vi "Eval y=f(a,x).vi"(4 "number of points":u32=10, 5 "formula":string, 6 "Parameters":cluster{"name":string, "value":dbl}[](array[cluster]) {"value" format="%.2f"}, 7 "end":dbl=1.0 format="%.2f", 8 "start":dbl format="%.2f") -> (0 "error":i32, 1 "ticks":u32, 2 "Y":dbl[](array[numeric]) format="%.2f", 3 "X":dbl[](array[numeric]) format="%.2f")   [LabVIEW 2020, in "NI_Gmath.lvlib"]
doc: "A generalized version of the Eval y=f(x) VI with the possibility of adding some parameters into the formula."
uses:
  <vilib>/gmath/NI_Gmath.lvlib
panel:
  # "Example:\n\n number of points: 100 \n start: 0.0\n end: 1.0\n Parameters: (a,1) and (b,2) \n formula: sin(t*a)+b"
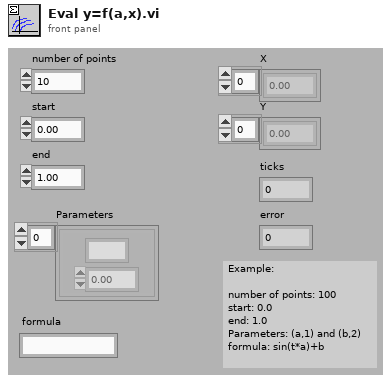
[diagram p1: front panel]
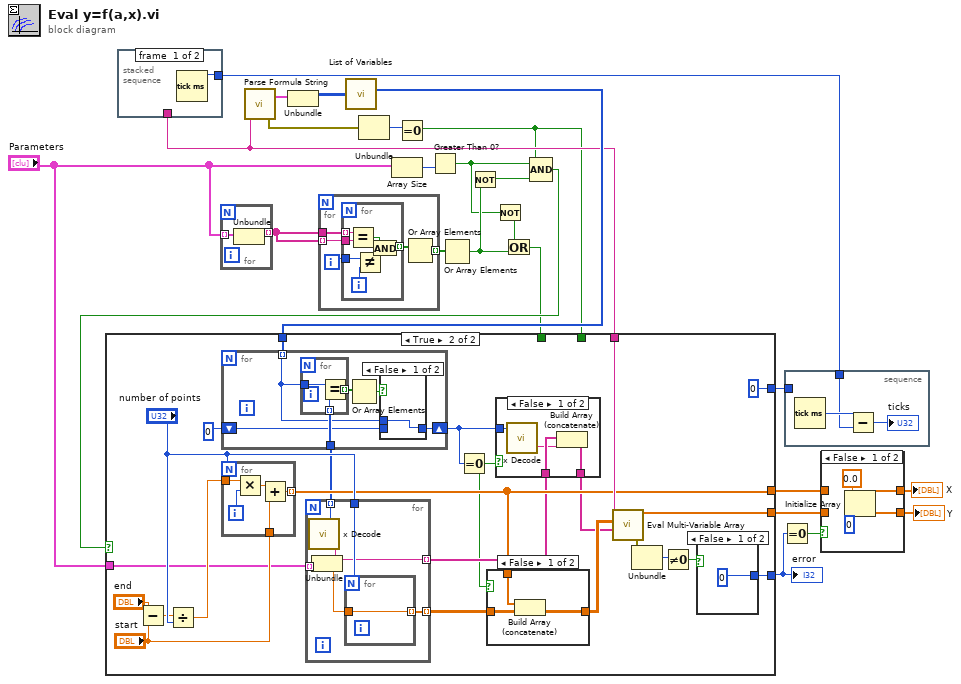
[diagram p0: block diagram]
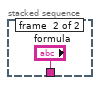
[diagram p3: hidden frame]
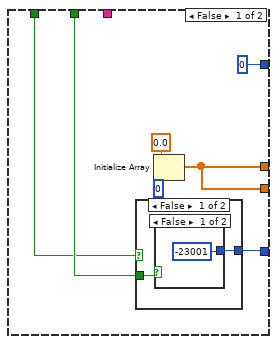
[diagram p4: hidden frame]
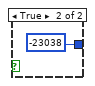
[diagram p5: hidden frame]
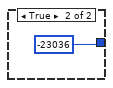
[diagram p6: hidden frame]
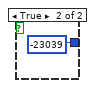
[diagram p10: hidden frame]
diagram:
  n1 = stacked-sequence {
    tunnel: [w26 _] -> w24
    tunnel: [_ "formula"] -> w4
    frame #0 {
      n2 = Tick Count (ms)() -> (millisecond timer value=w26:u32)
    }
    frame #1 {
    }
  }
  n3 = for {
    tunnel: "Parameters" -> [w29] mode=indexing
    tunnel: [w28] -> w12 mode=indexing
    n4 = Unbundle(w29) -> ("name"=w28:string)  [unwired: 1 out]
  }
  n5 = call <vilib>:"Parse Formula String.vi"("formula"=w4) -> ("error out"=w23:errorcluster, "Parsed Formula"=w15:cluster{"Table":i32[][], "Y Values":dbl[]})  [unwired: 1 in]
  n6 = Unbundle(w15) -> ("Table"=w14:i32[][])  [unwired: 1 out]
  n7 = for {
    tunnel: w12 -> [w34]
    tunnel: w12 -> [w33] mode=indexing
    tunnel: [w30] -> w11 mode=indexing
    i -> [w32]
    n8 = for {
      tunnel: w34 -> [w41] mode=indexing
      tunnel: w33 -> [w40]
      tunnel: w32 -> [w39]
      tunnel: [w35] -> w31 mode=indexing
      i -> [w38]
      n9 = Equal?(x=w41, y=w40) -> (x = y?=w37:bool)
      n10 = Not Equal?(x=w39, y=w38) -> (x != y?=w36:bool)
      n11 = And(x=w37, y=w36) -> (x .and. y?=w35:bool)
    }
    n12 = Or Array Elements(Boolean array=w31) -> (logical OR=w30:bool)
  }
  n13 = call <vilib>:"List of Variables.vi"("Table"=w14) -> ("List of variables"=w13:i32[])
  n14 = Unbundle(w23) -> ("code"=w22:i32)  [unwired: 2 out]
  n15 = Array Size(array="Parameters") -> (size(s)=w9:i32)
  n16 = Equal To 0?(x=w22) -> (x = 0?=w3:bool)
  n17 = Greater Than 0?(x=w9) -> (x > 0?=w7:bool)
  n18 = Or Array Elements(Boolean array=w11) -> (logical OR=w8:bool)
  n19 = Not(x=w8) -> (.not. x?=w10:bool)
  n20 = Not(x=w7) -> (.not. x?=w5:bool)
  n21 = Or(x=w5, y=w8) -> (x .or. y?=w2:bool)
  n22 = Compound Arithmetic op=AND(w3, w7, w10) -> (w6:bool)
  n23 = case shown="True" w6 {
    tunnel: w4 -> [_ w76]
    tunnel: [w45 w69] -> w19
    tunnel: [w45 w68] -> w17
    tunnel: [0 0] -> w25
    tunnel: [w44 w62] -> w21
    tunnel: w13 -> [_ w61]
    tunnel: "Parameters" -> [_ w58]
    tunnel: w3 -> [w43 _]
    tunnel: w2 -> [w42 _]
    frame False {
      n24 = case shown="False" w42 {
        tunnel: [w50 -23036] -> w44
        tunnel: w43 -> [w49 _]
        frame False {
          n25 = case shown="False" w49 {
            tunnel: [-23001 -23038] -> w50
            frame False {
            }
            frame True {
            }
          }
        }
        frame True {
        }
      }
      n26 = Initialize Array(0.0, 0) -> (w45:dbl[])
    }
    frame True {
      n27 = Subtract(x="end", y="start") -> (x-y=w70:dbl)
      n28 = Divide(x=w70, y="number of points") -> (x/y=w71:dbl)
      n29 = for {
        N: "number of points" -> [_]
        tunnel: w71 -> [w103]
        tunnel: "start" -> [w99]
        tunnel: [w100] -> w69 mode=indexing
        i -> [w102]
        n30 = Multiply(x=w103, y=w102) -> (x*y=w101:dbl)
        n31 = Add(x=w101, y=w99) -> (x+y=w100:dbl)
      }
      n32 = for {
        tunnel: w58 -> [w109] mode=indexing
        tunnel: [w105] -> w57 mode=indexing
        tunnel: "number of points" -> [w108]
        tunnel: [w106] -> w75 mode=indexing
        tunnel: [w104] -> w60 mode=indexing
        n33 = Unbundle(w109) -> ("name"=w105:string, "value"=w107:dbl)
        n34 = call <vilib>:"x Decode.vi"("x string"=w105) -> ("number"=w104:i32)  [unwired: 1 in, 1 out]
        n35 = for {
          N: w108 -> [_]
          tunnel: [w110] -> w106 mode=indexing
          tunnel: w107 -> [w110]
        }
      }
      n36 = for {
        tunnel: w61 -> [w86] mode=indexing
        tunnel: w60 -> [w91]
        shift-right: [w87] -> w54
        shift-left: 0 -> [w88]
        n37 = for {
          tunnel: w91 -> [w94] mode=indexing
          tunnel: w86 -> [w96]
          tunnel: [w95] -> w90 mode=indexing
          n38 = Equal?(x=w96, y=w94) -> (x = y?=w95:bool)
        }
        n39 = Or Array Elements(Boolean array=w90) -> (logical OR=w89:bool)
        n40 = case shown="False" w89 {
          tunnel: w88 -> [_ w93]
          tunnel: [w92 w93] -> w87
          tunnel: w86 -> [w92 _]
          frame False {
          }
          frame True {
          }
        }
      }
      n41 = Equal To 0?(x=w54) -> (x = 0?=w56:bool)
      n42 = case shown="False" w56 {
        tunnel: [w79 w80] -> w66
        tunnel: w69 -> [w78 _]
        tunnel: w75 -> [w77 w80]
        frame False {
          n43 = Build Array (concatenate)(w78, w77) -> (w79:dbl[][])
        }
        frame True {
        }
      }
      n44 = case shown="False" w56 {
        tunnel: w57 -> [w84 w85]
        tunnel: w54 -> [w83 _]
        tunnel: [w81 w85] -> w55
        frame False {
          n45 = call <vilib>:"x Decode.vi"("number"=w83) -> ("x string"=w82:string)  [unwired: 1 in, 1 out]
          n46 = Build Array (concatenate)(w82, w84) -> (w81:string[])
        }
        frame True {
        }
      }
      n47 = call <vilib>:"Eval Multi-Variable Array.vi"("Variables"=w55, "X Values"=w66, "formula"=w76) -> ("error out"=w65:errorcluster, "Y Values"=w68:dbl[])  [unwired: 1 in]
      n48 = Unbundle(w65) -> ("code"=w63:i32)  [unwired: 2 out]
      n49 = Not Equal To 0?(x=w63) -> (x != 0?=w64:bool)
      n50 = case shown="False" w64 {
        tunnel: [0 -23039] -> w62
        frame False {
        }
        frame True {
        }
      }
    }
  }
  "error" <- w21
  n51 = Equal To 0?(x=w21) -> (x = 0?=w20:bool)
  n52 = stacked-sequence {
    tunnel: w25 -> [_]
    tunnel: w24 -> [w111]
    frame #0 {
      n53 = Tick Count (ms)() -> (millisecond timer value=w112:u32)
      n54 = Subtract(x=w112, y=w111) -> (x-y=→"ticks":u32)
    }
  }
  n55 = case shown="False" w20 {
    tunnel: w19 -> [_ w118]
    tunnel: [w114 w118] -> w18
    tunnel: w17 -> [_ w117]
    tunnel: [w114 w117] -> w16
    frame False {
      n56 = Initialize Array(0.0, 0) -> (w114:dbl[])
    }
    frame True {
    }
  }
  "X" <- w18
  "Y" <- w16
